vi "Write Active Axis.vi"(8 "error in":errorcluster, 10 "Axis":T1=enum."X", 11 "Axis in":refnum<class "Axis.lvclass">) -> (0 "error out":errorcluster, 3 "Axis out":refnum<class "Axis.lvclass">)   [LabVIEW 2018, in "Axis.lvlib" / "Axis.lvclass"]
uses:
  Axis.lvclass
  Custom Controls/Axis.ctl
  Axis.lvclass/Axis.ctl
  Axis.lvlib
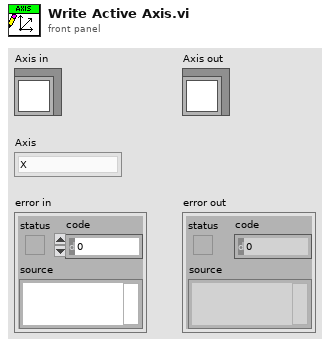
[diagram p1: front panel]
types:
  T1 = typedef "Axis.lvlib/Axis.ctl" = enum16{"None", "X", "Y", "Z", "Rx", "Ry", "Rz"}
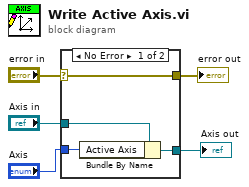
[diagram p0: block diagram]
diagram:
  n1 = case shown="No Error" "error in" {
    selector: "error in" -> [w9 w10]
    tunnel: [w9 w10] -> w4
    tunnel: [w7 w11] -> w2
    tunnel: "Axis in" -> [w8 w11]
    tunnel: "Axis" -> [w6 _]
    frame No Error {
      n2 = Bundle By Name(cluster=w8, "Active Axis"=w6) -> (w7:refnum<class "Axis.lvclass">)
    }
    frame Error {
    }
  }
  "error out" <- w4
  "Axis out" <- w2
